vi "KI6221.vi"() -> ()   [LabVIEW 2025]
uses:
  Instance          14 14Saved   KI6221 .vi
  Instance          66 14Saved   KI6221 .vi
  Instance          40 14Saved   KI6221 .vi
  Instance          41 14Saved   KI6221 .vi
  Instance          42 14Saved   KI6221 .vi
  Instance          45 14Saved   KI6221 .vi
  Instance          50 14Saved   KI6221 .vi
  Instance          61 14Saved   KI6221 .vi
  Instance          62 14Saved   KI6221 .vi
  Instance          60 14Saved   KI6221 .vi
  Instance          68 14Saved   KI6221 .vi
  Instance          67 14Saved   KI6221 .vi
  Instance          51 14Saved   KI6221 .vi
  Instance          52 14Saved   KI6221 .vi
  Instance          53 14Saved   KI6221 .vi
  Instance          57 14Saved   KI6221 .vi
  Instance          55 14Saved   KI6221 .vi
  Instance          56 14Saved   KI6221 .vi
  Instance          54 14Saved   KI6221 .vi
  Instance          65 14Saved   KI6221 .vi
  Instance          64 14Saved   KI6221 .vi
  Instance          63 14Saved   KI6221 .vi
  Instance          37 14Saved   KI6221 .vi
  Instance          36 14Saved   KI6221 .vi
  Instance          35 14Saved   KI6221 .vi
  Instance          34 14Saved   KI6221 .vi
  Instance          39 14Saved   KI6221 .vi
  Instance          38 14Saved   KI6221 .vi
  Instance          49 14Saved   KI6221 .vi
  Instance          48 14Saved   KI6221 .vi
  Instance          43 14Saved   KI6221 .vi
  Instance          44 14Saved   KI6221 .vi
  Instance          31 14Saved   KI6221 .vi
  Instance          30 14Saved   KI6221 .vi
  Instance          32 14Saved   KI6221 .vi
  Instance          29 14Saved   KI6221 .vi
  Instance          33 14Saved   KI6221 .vi
  Instance          47 14Saved   KI6221 .vi
  Instance          26 14Saved   KI6221 .vi
  Instance          27 14Saved   KI6221 .vi
  Instance          28 14Saved   KI6221 .vi
  Instance           6 14Saved   KI6221 .vi
  Instance           5 14Saved   KI6221 .vi
  Instance           7 14Saved   KI6221 .vi
  Instance          11 14Saved   KI6221 .vi
  Instance          12 14Saved   KI6221 .vi
  Instance          13 14Saved   KI6221 .vi
  Instance          23 14Saved   KI6221 .vi
  Instance          22 14Saved   KI6221 .vi
  Instance          21 14Saved   KI6221 .vi
  Instance          20 14Saved   KI6221 .vi
  Instance          19 14Saved   KI6221 .vi
  Instance          46 14Saved   KI6221 .vi
  Instance          25 14Saved   KI6221 .vi
  Instance          18 14Saved   KI6221 .vi
  Instance          17 14Saved   KI6221 .vi
  Instance           3 14Saved   KI6221 .vi
  Instance           4 14Saved   KI6221 .vi
  Instance           2 14Saved   KI6221 .vi
  Instance          10 14Saved   KI6221 .vi
  Instance           9 14Saved   KI6221 .vi
  Instance           8 14Saved   KI6221 .vi
  <vilib>/Utility/file.llb/Write To Spreadsheet File (DBL).vi
  Instance          15 14Saved   KI6221 .vi
  Instance          16 14Saved   KI6221 .vi
  Instance          24 14Saved   KI6221 .vi
  <vilib>/express/express arith-compare/Formula/XNode/ExpressFormulaBlockNode.xnode
panel:
  in  "Case Constant\n(See Context Help) 9":bool=TRUE
  in  "Case Constant\n(See Context Help) 8":bool
  in  "Case Constant\n(See Context Help) 7":bool=TRUE
  in  "Case Constant\n(See Context Help) 6":bool=TRUE
  in  "Case Constant\n(See Context Help) 5":bool
  in  "Case Constant\n(See Context Help) 4":bool=TRUE
  in  "Case Constant\n(See Context Help) 3":bool
  in  "Case Constant\n(See Context Help) 2":bool
  in  "Case Constant\n(See Context Help)":bool=TRUE
  in  "last amp":string="*.txt"
  in  "init":bool=TRUE
  out "error out 38":errorcluster
  out "error out 37":errorcluster
  out "auto test label":string="                                                               Auto-Test Sequence Running\nThe Auto-Test sequence is attempting to locate the corresponding current levels for the voltage endpoints selected. Please be patient. If correct values can not be located, a warning window will appear. That would usually mean that either the device connections are incorrect, there is not enough signal to accurately locate the source points, or something other than the current sourced may effecting the voltage measurment."
  out "demo warning":string="DEMO MODE ON! DATA IS NOT LIVE!"
  out "INCREMENT":dbl
  in  "nv METER LAST":u16=5
  in  "enable measure LAST":bool=TRUE
  out "error out 36":errorcluster
  out "Default path 2":path=path "C:/6220software/data"
  in  "CONNECT\nONLY FLAG":bool
  in  "CAP LAST":bool
  in  "H,L,G Haz volt LAST":bool
  in  "Nearby AC voltages LAST":bool
  out "error out 35":errorcluster
  out "error out 31":errorcluster
  out "error out 22":errorcluster
  in  "Y Axis:  LAST":u16(ring)=3 items=["Points", "Time", "Current", "Voltage", "Resistance"]
  in  "X Axis: LAST":u16(ring) items=["Points", "Time", "Current", "Voltage", "Resistance"]
  out "error out 19":errorcluster
  out "error out 18":errorcluster
  in  "Source TABS LAST":u32=99
  out "error":errorcluster
  in  "Activate Output LAST":bool
  in  "Current Source \nVoltage Compliance (V) LAST":dbl=10.01 min=0.1 max=105.0 step=0.01 format="%^#_6g"
  in  "Source Level (Amps) LAST":dbl min=-0.105 max=0.105 format="%^#_9e"
  in  "SUM LAST":i32=7
  in  "NEXT FLAG LAST":i32=-1
  in  "NEXT FLAG":i32
  in  "SETUP FLAG":i32=1
  in  "Main Tabs":T1(tab)=enum."Basic Operation"
  in  "COMM\nTab Control":T2(tab)
  in  "EXIT 2":bool
  in  "conn guide":bool
  in  "SAVE 2":bool
  in  "OPEN":bool
  in  "Test file description and comments:":string="Enter details to remember about this test here. It will be saved with your test file."
  in  "EDIT present setup":bool
  in  "NEW INSTR SETUP":bool
  out "Current Test File:":path
  in  "CAP IN":u16(ring) caption="When using GUARDED CONNECTIONS we suggest that, when possible, a LO to EARTH \nConnection be made on the rear of the instrument. If this is possible given your test setup\nand goals make certain the box below is checked. If connecting instrument LO to EARTH for\nyour measurement is infeasible make certain the box below is not checked.\n         *NOTE: This response effects only how the instrument is setup. \n           Fundamentally, the measurement can be made either way." items=["NORMAL OPERATION", "REDUCE C IN 2182A"]
  in  "CANCEL":bool
  in  "BACK":bool
  out "Main intro bar":picture
  out "instrument status":string="SETUP UNVERIFIED"
  in  "Verify instruments":bool
  in  "connect HELP LINK":bool
  in  "LOW to EARTH 2":u16(ring) caption="When using GUARDED CONNECTIONS we suggest that, when possible, a LO to EARTH \nConnection be made on the rear of the instrument. If this is possible given your test setup\nand goals make certain the box below is checked. If connecting instrument LO to EARTH for\nyour measurement is infeasible make certain the box below is not checked.\n         *NOTE: This response effects only how the instrument is setup. \n           Fundamentally, the measurement can be made either way." items=["NO  EARTH  CONNECTION IN SOURCE", "LO TO EARTH CONNECTION"]
  in  "Power:":u16(ring) items=["60 Hz", "50 Hz"]
  in  "default use 2":bool
  in  "DEFAULT setup":bool=TRUE
  in  "OK":bool
  in  "HI IMP devices?":u16(ring) caption="Hi Impedance Devices also make voltage measurements more difficult. Since the input \nimpedance of the 2182 is about 10 GOhms you can approximate the 'loading error' by \ntaking your device impedance and dividing by 10^7. Therefore, if your device impedance is\n10 MOhm, then your loading error is 0.001 or 0.1%.You can compensate for this by using\nCONNECTIONS FOR HI IMPEDANCE DEVICES, however the trade off is that your noise floor\nincreases to about 100 nV RMS using this connection scheme because of the buffered input." items=["4-WIRE CONNECTIONS TO DUT", "2-WIRE CONNECTIONS TO DUT"]
  in  "6220 Connect":u16(ring)=1 caption="The current source is set up for easy cabling in STANDARD CONNECTIONS mode. This \nallows for many versatile measurement setups. However, with high impedance\ndevices or with significant cable capacitance the RC product in the circuit can impact the \ninstrument's risetime for some tests. If you would like to make GUARDED CONNECTIONS\nbecause of the RC present in your test system or for any other reason select GUARDED\nCONNECTIONS below, otherwise use STANDARD CONNECTIONS." items=["SELECT", "UNGUARDED SOURCING", "GUARDED SOURCING"]
  in  "Select GPIB Board number:\n(default to zero)":i32 min=0 max=7
  in  "Select GPIB Address number \nof the current source:":i32=16 min=0 max=32
  out "GPIB 6220 label":string="The 6220 must be connected in GPIB mode. Select the settings below."
  in  "Select Network Card number:\n(default to zero)":i32 min=0 max=7
  in  ".  IP#4":i32=160 min=0 max=255 format="%03.0f"
  in  ".  IP#3":i32=27 min=0 max=255 format="%03.0f"
  in  ".  IP#2":i32=40 min=0 max=255 format="%03.0f"
  in  "Input instrument IP Address:":i32=10 min=0 max=255 format="%03.0f"
  in  "Select the interface for the 6220/6221:":u16(ring)=1 items=["SELECT", "ETHERNET", "GPIB"]
  in  "Select the nanovoltmeter model number:":u16(ring)=3 items=["SELECT", "NONE", "2182", "2182A"]
  in  "Select the current source model number:":u16(ring)=2 items=["SELECT", "6220", "6221"]
  in  "LOW to EARTH":bool caption="When using GUARDED CONNECTIONS we suggest that, when possible, a LO to EARTH \nConnection be made on the rear of the instrument. If this is possible given your test setup\nand goals make certain the box below is checked. If connecting instrument LO to EARTH for\nyour measurement is infeasible make certain the box below is not checked.\n         *NOTE: This response effects only how the instrument is setup. \n           Fundamentally, the measurement can be made either way."
  in  "Lo earth HELP":bool
  in  "Src Connect HELP":bool
  in  "DUT connect HELP":bool
  out "WIZ string":string="Instrument Communication Setup"
  in  "NEXT":bool
  in  "nVm C HELP":bool
  in  "Previous":bool
  in  "AC HELP":bool
  in  "HAZARD HELP":bool
  in  "4 step TABS":T3(tab)
  out "step 1 pic":picture
  out "step 2 pic":picture
  out "step 3 pic":picture
  out "step 4 pic":picture
  in  "CAP":bool
  in  "H,L,G Haz volt":bool caption="I need to shield my device because:"
  in  "Nearby AC voltages":bool
  in  "start of guide":bool
  in  "END OF GUIDE":bool
  in  "NEXT GUIDE":bool
  in  "RETURN TO SPLASH SCREEN":bool
  in  "setup wizard":bool
  in  "default use":bool
  in  ".  IP#4":i32=160 min=0 max=255 format="%03.0f"
  in  ".  IP#3 2":i32=27 min=0 max=255 format="%03.0f"
  in  ".  IP#2":i32=40 min=0 max=255 format="%03.0f"
  in  "at instrument IP Address:":i32=10 min=0 max=255 format="%03.0f"
  in  "at GPIB Address:":i32=16 min=0 max=32
  in  "Model 6220 or 6221 is connected by:":u16(ring) items=["Ethernet", "GPIB"]
  in  "GPIB Address:":i32=24 min=0 max=32
  in  "INSTRUMENT NAME:":string="2400"
  in  "step setup CANCEL":bool
  in  "step setup OK":bool
  in  "DELAY in mS":i32=20 min=0
  in  "GO TO LEVEL:                *NOTE - MUST include <LEVEL>":string=":sour:volt:lev <LEVEL>"
  in  "DEACTIVATE:":string=":outp:stat off"
  in  "CONFIGURE:":string="*rst\n:sour:func volt\n:outp:stat on"
  in  "RESPONSE STRING:":string="2400"
  in  "VERIFY:":string="*IDN?"
  out "TREE DIAGRAM":picture
  out "Step source setup directions":string="Step Source Setup\nTo configure your step source correctly you must identify the GPIB commands that must be sent at each step in the testing process. The tree below defines this process. In each space to the right enter the GPIB commands that need to be sent to your stepping instrument. Each section can contain zero, one, or many commands. Each command should be separated by a Carriage Return. Do not include quotation marks or any punctuation that you do not want sent directly to the instrument. Here is a description of each step in the test:\n\nINSTRUMENT NAME - Instrument name to appear in drop down menu. This is a REQUIRED FIELD.\n\nGPIB Address - The address setting of the step source instrument.\n\nVERIFY - This section simply tests to see if the instrument responds on the bus. For Keithley Instruments this would typically be a \"*idn?\". After this section of code a READ is automatically done by the software and the response is searched to see if it includes the RESPONSE STRING. If the response string does appear, then the instrument is said to be found. If there is no response or a response without the response string, then the instrument is not found.\n\nVerify example:    *idn?\nResponse string example:   2400\n\nCONFIGURE - These commands are sent only once just after a test is executed. It should setup the instrument and activate the source at some safe level.\n\nexample:            *rst\n                           :form:elem 'volt','curr'\n                           :sour:func curr\n                           :sour:curr:rang:auto on\n                           :outp:stat on\n\nGO TO LEVEL - These commands are run once per loop. They should only set the source to the appropriate bias level for the next sweep by the 6220 and 2182. You MUST use the input variable <LEVEL> in this code. This text will be replaced with the next bias level as set from the test screen. DELAY is the time in milliseconds for the program to wait between sending these commands to the bias instrument and beginning the next 6220/2182 sweep. Use this delay to allow the bias source and device to settle before the next sweep.\n\nGO TO LEVEL example:   :sour:curr:lev <LEVEL>\n\nDEACTIVATE - These commands should be used to deactivate the step source after the last sweep. This is important for test safety.\n\nDEACTIVATE example:   :outp:stat off\n\nDATA QUERY - This is the command that tells the instrument to return data. The type of data to be returned should be set up previously in the CONFIGURE section. This is a one line command usually ending in a ?. During execution it will be immediately followed by a read which will collect the data from the instrument.\n\nDATA QUERY example:     :trac:data?\n\nNumber and Names for data Returned - Correctly fill the blank strings with names for data that will be returned. I.E. If your step source will be returning voltage and current data  enter 'Voltage' in the string when number shows 0, then click up. Now that the number reads 1 type 'Current' in the string. Make sure the strings linked to 2 and above are blank. These inputs tell the program how many different types of data it will receive as well as what to name the data vectors on data sheets and graphs. Typically, the data points are Interleaved. This means that when the instrument sends the long string of data back it would read:\n\n(Voltage,Current,Voltage,Current,....)\n\nIf this were the case you would set the data names as above.\nThen set the Data Delimiter to , \nThe Data Prefix would be (\nThe Data Suffix would be )\nand the data is interleaved so the box would be checked.\n\nAnother example:\n\nInstruments will send back:\n\nVoltage;Voltage;Voltage;.......;Current;Current;Current;\n\nIn this case set the inputs like so:\n\nNumber and Name as above.\nData Prefix:   \nData Suffix:    ;\nData Delimiter:    ;\nData is Interleaved is NOT checked because all the voltage points appear before the current values.\n\nData Prefix is left blank because nothing appears before the first number. Data Suffix is set to ; because there is a semicolon after the last data point. Data Delimiter is also set to ; because a semicolon appears between each data point.\nIf you don't wish to return any data leave the DATA QUERY blank.\n\nWhen all of your commands are correctly set click OK below. Click CANCEL to exit without saving at any time.\n"
  in  "GENERATE SCPI - BASIC":bool
  in  "Basic Source":enum32{"DC Source", "DC Sweep", "AC Source"}(tab)=enum."DC Sweep"
  in  "TAKE CONTROL":bool
  in  "Current Source \nVoltage Compliance (V)":dbl=10.01 min=0.1 max=105.0 step=0.01 format="%^#_6g"
  in  "Activate Output":bool
  in  "Source Level (Amps)":dbl min=-0.105 max=0.105 step=1e-12 format="%^#_9e"
  in  "ABORT SWEEP":bool
  in  "RUN SWEEP":bool
  in  "delta tabs 2":enum32{"GRAPH", "SHEET"}(tab)
  in  "Y Axis:":u16(ring)=3 items=["Points", "Current", "Voltage", "Resistance"]
  in  "X Axis:":u16(ring) items=["Points", "Current", "Voltage", "Resistance"]
  out "I Sweep Graph":cluster{"Y":dbl[], "Y":dbl[]}[](graph)
  out "I Sweep V Measure Data":string[][](table)
  in  "basic sweep tabs":enum32{"Source", "Measure"}(tab)
  in  "Delay (settle time in sec)":dbl=0.01 min=0.001 max=9999000.0 format="%^#_6g"
  in  "Sweep Type":u16(ring) items=["Linear ", "Logarithmic"]
  in  "Current Source \nVoltage Compliance (V)":dbl=10.0 min=0.1 max=105.0 step=0.01 format="%^#_6g"
  in  "Stop Current (Amps)":dbl=0.005 min=-0.105 max=0.105 format="%^#_6g"
  in  "Number of sweep points":i32=50 min=2 max=65536
  in  "Start Current (Amps)":dbl=0.001 min=-0.105 max=0.105 format="%^#_6g"
  in  "Measurement Integration \n(NPLCs)":dbl(ring)=1.0 items=["0.01"=0.01, "0.1"=0.1, "1"=1.0, "10"=10.0]
  in  "enable measure":bool=TRUE
  in  "Voltage Measure Range":dbl(ring)=0.1 items=["10 mV"=0.01, "100 mV"=0.1, "1 V"=1.0, "10 V"=10.0, "100 V"=100.0]
  in  "STOP 2":bool
  in  "RUN 2":bool
  in  "Voltage\n Compliance":dbl=10.0 min=0.1 max=105.0 step=0.01 format="%#_3f"
  in  "Signal Repetition \nFrequency (Hz)":dbl=10.0 min=0.0001 max=100000.0 format="%.4f"
  in  "Waveform Type":u16(ring)=1 items=["RAMP", "SQUARE", "SINE"]
  in  "waveform tabs 2":enum32{"RAMP", "SQUARE", "SINE"}(tab)=enum."SQUARE"
  in  "Duty Cycle (%)":dbl=50.0 min=0.0 max=100.0 format="%#.2f"
  in  "Ramp to: (Amps)":dbl min=-0.105 max=0.105 step=1e-12 format="%^#_6g"
  in  "Ramp from: (Amps)":dbl min=-0.105 max=0.105 step=1e-12 format="%^#.6g"
  in  "Duty Cycle (%)":dbl=50.0 min=0.0 max=100.0 format="%#.2f"
  in  "Offset (Amps)":dbl min=-0.105 max=0.105 step=1e-12 format="%^#_6g"
  in  "Amplitude (Amps)":dbl=0.105 min=0.0 max=0.105 step=1e-12 format="%^#.6g"
  in  "Offset (Amps)":dbl=0.01 min=-0.105 max=0.105 step=1e-12 format="%^#.6g"
  in  "Amplitude (Amps)":dbl=2e-12 min=2e-12 max=0.105 step=1e-12 format="%^#_6g"
  in  "GENERATE SCPI - ADVANCED":bool
  in  "Advanced Operation Tab":T4(tab)=enum."ARB Waveform Generator"
  in  "SAVE DELTA DATA":bool
  in  "CLEAR DELTA DATA":bool
  in  "delta tabs":enum32{"GRAPH", "SHEET", "HELP"}(tab)=enum."HELP"
  in  "Y Axis:":u16(ring) items=["Resistance", "Delta Voltage", "Conductance", "Power"]
  in  "X Axis:":u16(ring) items=["Points", "Time"]
  out "Delta Mode Resistance Graph":cluster{"Y":dbl[], "Y":dbl[]}[](graph)
  out "Delta Mode Measurement Data":string[][](table)
  out "Delta Measurements\nHelp":string="Delta Mode measurements are typically used on low resistance devices where noise from thermal electromotive forces becomes an issue. This software sets up an alternating current source with coordinated voltage measurements that can help to cancel out these noise sources. The inputs for this measurement are explained here:\n\nOn the Setup Tab:\n\nHigh Current (Amps) - This is the higher current value that the source will alternate between.\n\nLow Current (Amps) - This is the lower of the two alternating current values.\n\nNumber of cycles - This is the number of cycles that will be run during the test. \n\nFiltering - For Delta Mode measurements the instruments can implement either a moving filter (which averages the last X number of readings like a rolling filter) or a Repeat Filter (which only reports a result after X new readings are averaged). The number of readings is set by Filter Count. When no filter is selected Filter Count is disregarded.\n\nVoltage Measure Range - The range setting on the nanovoltmeter. A fixed range must be selected for delta mode measurements. \n\n_______________________\n\nOn the Advanced Tab:\n\nDelay (mS) - This is the delay time between the setting of the current value and the beginning of the measurement integration on the nanovoltmeter.\n\nMeasurement Integration (NPLCs) - This is the integration time for the nanovoltmeter expressed in Number of Power Line Cycles. On 60 Hz power a cycle represents 16.667 milliseconds. The lowest noise from the nanovoltmeter tends to be between 2 and 4 NPLCs for delta measurements.\n\nCurrent Source Voltage Compliance - This is the maximum potential created across the current source output leads. This should be set depending on safety and the fragility of the devices under test. This limit can be exceeded for a few microseconds until the 622X can respond. See the manual for more details.\n\nDelta Demo Mode - The demo mode button displays the demo graph for viewing example data and taking new data to show the difference between DC and Delta mode resistance measurements.\n\nAfter Run is clicked the Data Sheet and the graph will fill with data points as they are collected. The point number, delta voltage readings, the calculated resistance, the calculated conductance, the calculated power, and time stamp are all recorded. Use the X and Y Axis controls to alter the graph. Power will not be calculated if the delta is not centered around 0 (Zero DC Power)."
  out "DELTA DIAGRAM":picture
  in  "DELTA HELP LINK":bool
  in  "Guide help 3":bool
  in  "delta user tabs":enum32{"SETUP", "ADVANCED"}(tab)
  in  "Filter\nCount":i32=50 min=2 max=300
  in  "FILTER":u16(ring)=1 items=["NO Filter", "Moving Filter", "Repeat Filter"]
  in  "Voltage Measure Range":dbl(ring)=0.01 items=["10 mV"=0.01, "100 mV"=0.1, "1 V"=1.0, "10 V"=10.0, "100 V"=100.0]
  in  "INFINITE DELTA CYCLES":bool
  in  "Number of Readings":i32=1000 min=1 max=65536
  in  "Low Current (Amps)":dbl=-0.0004 min=-0.105 max=0.105 format="%^#_8e"
  in  "High Current (Amps)":dbl=0.0004 min=-0.105 max=0.105 format="%^#_8e"
  in  "DELTA DEMO":bool
  in  "DAMPING":bool
  in  "Current Source \nVoltage Compliance (V)":dbl=10.0 min=0.1 max=105.0 step=0.01 format="%^#_6g"
  in  "Measurement Integration (NPLCs)":dbl=1.0 min=1.0 max=50.0 step=1.0 format="%#_4f"
  in  "Current Source Range":dbl(ring) items=["BEST FIXED"=0.0, "100 mA"=0.1, "20 mA"=0.02, "2 mA"=0.002, "200 uA"=0.0002, "20 uA"=2e-05, "2 uA"=2e-06, "200 nA"=2e-07, "20 nA"=2e-08, "2 nA"=2e-09]
  in  "Delay (mS) - settle time":dbl=1.0 min=1.0 max=9999000.0 format="%^#_6g"
  in  "ABORT DELTA":bool
  in  "RUN DELTA":bool
  in  "DC TABS":enum32{"2-D GRAPH", "3-D PLOT", "SHEET", "HELP"}(tab)=enum."HELP"
  out "Differential Conductance Graph":cluster{"Y":dbl[], "Y":dbl[]}[](graph)
  in  "Vertical Axis:":u16(ring)=2 items=["Delta Voltage", "Resistance", "Conductance"]
  in  "Horizontal Axis:":u16(ring) items=["Voltage", "Current"]
  in  "Differential Conductance Surface Plot":refnum<k7>(container)
  in  "Plot reset":bool
  in  "Plot style":i32(ring)=5 items=["cwLine"=1, "cwPoint"=2, "cwLinePoint"=3, "cwHiddenLine"=4, "cwSurface"=5, "cwSurfaceLine"=6, "cwSurfaceNormal"=7, "cwContourLine"=8, "cwSurfaceContour"=9]
  in  "Transparency (%)":dbl(knob) scale=0.0..90.0
  in  "Projection":bool
  out "Differential Conductance Measurement Data":string[][](table)
  out "DIFF COND DIAGRAM":picture
  out "Differential Conductance \nHelp":string="Differential Conductance sweeps can be controlled in several different ways and the results examined through a number of graphs or charts.\n\nFirst, a discussion of the inputs that define a single differential conductance sweep:\n\nOn the Setup Panel:\n\nWhen controlling the sweep in terms of current these inputs appear:\n\nStart Current (Amps) - the first current value to generate a conductance reading.\n\nStop Current (Amps) - the last current value to generate a reading.\n\nNumber of sweep points - the number of points including start and stop to return values. I.E. if start is -1 nA and stop is 1 nA and number of sweep points is 21, then the first reading is taken at -1 nA, then -900 pA, -800 pA, -700 pA,.....900 pA, 1 nA.\n\nVoltage Measure Range - The range setting on the nanovoltmeter. A fixed range must be selected for Differential Conductance sweeps.\n________________________________________\n\nWhen controlling the sweep in terms of voltage these inputs appear:\n\nStart Voltage (mV) - the first voltage value to generate a conductance reading.\n\nStop Voltage (mV) - the last voltage value to generate a reading.\n\nNumber of sweep points - the number of points including start and stop to return values. I.E. if start is -1 mV and stop is 1 mV and number of sweep points is 21, then the first reading is taken at -1 mV, then -900 uV, -800 uV, -700 uV,.....900 uV, 1 mV.\n\nWhen defining the test in terms of voltage there is one other input that is enabled on the Advanced Tab. Because the test is actually being conducted by a current source and voltmeter the voltages need to be related to current. The user can select to estimate the device resistance and the instrument will convert the data points using Ohm's Law. This will work for single sweeps, but if the step source is being used to conduct multiple sweeps and create a 3-D graph, then the disadvantage is that the  start and end points may not line up appopriately as the device resistance changes at different bias points. If this is a concern then the Auto Test is recommended. Auto-Test conducts a search to find the correct voltage endpoints at the beginning of each sweep.\n\nVoltage Measure Range - This is selected automatically when controlling in voltage mode. The control will be disabled.\n\nCurrent Source Voltage Compliance - Thsi control appears on the Advanced Tab but is disabled when in voltage mode just like the Voltage Measure Range.  This is the maximum potential created across the current source output leads. This should be set depending on safety and the fragility of the devices under test. This limit can be exceeded for a few microseconds until the 622X can respond. See the manual for more details.\n_________________________________________\n\nOnly available on the Advanced Tab in Current controlled mode:\n\nCurrent Source Voltage Compliance -  This is the maximum potential created across the current source output leads. This should be set depending on safety and the fragility of the devices under test. This limit can be exceeded for a few microseconds until the 622X can respond. See the manual for more details.\n_________________________________________\n\nWhichever way you control the test these parameters must also be selected from the Advanced Tab:\n\nMeasurement Integration (NPLCs) - This is the integration time for the nanovoltmeter expressed in \nNumber of Power Line Cycles. On 60 Hz power a cycle represents 16.667 milliseconds. The lowest noise from the nanovoltmeter tends to be between 2 and 4 NPLCs for delta measurements.\n\nFiltering - For Differential Conductance measurements a Repeat Filter (which only reports a result after X new readings are averaged) can be used. The number of readings is set by Filter Count. Selecting NO Filter will disable the filter and the filter count will be ignored.\n\nDelay (settle time in mS) - this is the wait time between when the current step is made and the integration of the voltage measurement begins to allow for settling of the circuit. This is expressed in milliseconds. 1 msec is the minimum delay.\n___________________________________________\n\nFor conducting multiple differential conductance sweeps access the Step Setup Tab.\n\nEnable the step setup functions by checking the enable step source checkbox.\nOnce the step source is enabled, select start, stop, and number of step values for that source are enabled.\n\nThe Trace Offset (%Pk-Pk) control sets the y-axis offset between multiple sweeps (for the 2-D Graph), so the user can adjust how they overlap.\n\nIf the step source is disabled, one sweep will be run.\n\nUse the RUN and ABORT buttons directly below to control the test execution.\n\n"
  in  "DC HELP LINK":bool
  in  "Guide help 1":bool
  in  "DC user tabs":enum32{"SETUP", "ADVANCED", "STEP SE"}(tab)
  in  "I want to control my test in terms of:":u16(ring)=1 items=["Voltage", "Current"]
  in  "V or I DIFF CON tabs":enum32{"Voltage", "Current"}(tab)=enum."Current"
  out "voltage message":string="Voltage source compliance\nand measure range will be set automatically."
  in  "Stop Voltage (Volts)":dbl=0.1 min=-100.0 max=100.0 step=0.005 format="%^#_8g"
  in  "Number of sweep points":i32=101 min=2 max=65536
  in  "Start Voltage  (Volts)":dbl min=-100.0 max=100.0 format="%^#_8g"
  in  "Stop Current (Amps)":dbl=0.001 min=-0.105 max=0.105 format="%^#_6g"
  in  "Number of sweep points":i32=101 min=2 max=65536
  in  "Start Current (Amps)":dbl=-0.001 min=-0.105 max=0.105 format="%^#_6g"
  in  "Voltage Measure Range":dbl(ring)=0.01 items=["10 mV"=0.01, "100 mV"=0.1, "1 V"=1.0, "10 V"=10.0, "100 V"=100.0]
  in  "Delay (settle time in mS)":dbl=2.0 min=1.0 max=9999000.0 format="%^#_6g"
  in  "FILTER":u16(ring) items=["NO Filter", "Repeat Filter"]
  in  "Resistance in Ohms":dbl=100.0 min=1e-07 max=10000000000.0 format="%^#_6g"
  in  "Define source points with an:":u16(ring) items=["Auto-Test", "Estimated Resistance"]
  in  "Repeat Filter Count:":i32=2 min=2 max=300
  in  "DIFF COND DAMPING":bool
  in  "Measurement Integration (NPLCs)":dbl=1.0 min=1.0 max=50.0 step=1.0 format="%#_2f"
  in  "Current Source \nVoltage Compliance (V)":dbl=10.0 min=0.1 max=105.0 step=0.01 format="%^#_6g"
  in  "DELETE SOURCE":bool
  in  "Trace offset (% Pk-Pk):":dbl
  in  "HELP":bool
  in  "edit commands STEP SOURCE":bool
  in  "Select step source:":u16(ring) items=["2400", "Window Pop-up", "NONE", "NEW..."]
  in  "Enable \nSTEP SOURCE":bool=TRUE caption="Enable step source"
  in  "Number of steps":i32=100 min=1
  in  "Stop Level":dbl=1.0 format="%^#_3e"
  in  "Start Level":dbl format="%^#_3e"
  in  "DIFF COND SAVE DATA":bool
  in  "CLEAR DATA DIFF COND":bool
  in  "ABORT DIFF COND":bool
  in  "RUN DIFF COND":bool
  in  "PULSE user tabS":enum32{"SETUP", "TIMING", "ADVANCED"}(tab)
  in  "Voltage Measure Range":dbl(ring)=0.01 items=["10 mV"=0.01, "100 mV"=0.1, "1 V"=1.0, "10 V"=10.0, "100 V"=100.0]
  in  "Pulse Mode:":u16(ring)=1 items=["Sweep Pulse Amplitude", "Repeat Pulse Amplitude"]
  in  "PULSE SWEEP OR LEVEL TABS":enum32{"Sweep", "Repeat"}(tab)
  in  "Number of Pulses":i32=101 min=2 max=65536
  in  "Sweep Type":u16(ring) items=["Linear ", "Logarithmic"]
  in  "Stop Pulse Level (Amps)":dbl=0.05 min=-0.1 max=0.1 format="%^#_3e"
  in  "Start Pulse Level (Amps)":dbl min=-0.1 max=0.1 format="%^#_3e"
  in  "Pulse Filter Count":i32=2 min=2 max=300
  in  "PULSE FILTER":u16(ring) items=["NO Filter", "Moving Filter", "Repeat Filter"]
  in  "INFINITE REPEAT PULSE CYCLES":bool
  in  "Number of Readings":i32=100 min=1 max=65536
  in  "Pulse Level (Amps)":dbl=0.01 min=-0.105 max=0.105 format="%^#_6g"
  in  "Pulse Width (mS)":dbl=0.05 min=0.05 max=12.0 step=0.001 format="%^#.3g"
  in  "Interval between Pulses (NPLC)":dbl=5.0 min=5.0 max=999990.0 step=1.0 format="%^#_10g"
  in  "Delay - pulse settle time in mS":dbl=0.016 min=0.016 max=11.966 step=0.001 format="%^#.4g"
  in  "Number of Pulse Off Measurements":i32=2 min=0 max=2 step=1
  in  "Pulse Off Level (Amps)":dbl min=-0.105 max=0.105 format="%^#_6g"
  in  "Current Source \nVoltage Compliance (V)":dbl=10.0 min=0.1 max=105.0 step=0.01 format="%^#_3g"
  in  "pulse TABS":enum32{"GRAPH", "SHEET", "HELP"}(tab)=enum."HELP"
  in  "Y Axis:":u16(ring) items=["Resistance", "Voltage", "Conductance", "Power", "Average Power"]
  in  "X Axis:":u16(ring) items=["Points", "Current", "Time"]
  out "Pulsed IV Graph":cluster{"Y":dbl[], "Y":dbl[]}[](graph)
  out "PULSE DATA SHEET":string[][](table)
  in  "PULSE HELP BUTTON":bool
  in  "PULSE HELP TABS":enum32{"DIAGRAM 2", "DIAGRAM"}(tab)=enum."DIAGRAM"
  out "PULSE DIAGRAM-SWEEP":picture
  out "PULSE DIAGRAM":picture
  out "Pulsed IV Measurements \nHelp":string="The Model 6221 Current Source uses a special pulse mode to coordinate with the Model 2182A. These pulses can then be used to collect current and voltage data for many devices, especially those with power limitations.\n\nFrom the setup tab you can select either sweep pulse mode or repeat pulse mode. In sweep pulse mode enter the start and stop value for the pulse as well as a number of pulses and a sweep type  which set a linear or logarithmic sweep function. In repeat pulse mode set the pulse level (Amps) and the number of pulses. Set the voltage measurement range for the nanovoltmeter for the highest range you will need whether you are repeating or sweeping pulses.\n\nOn the timing tab set the pulse width (ms) and a delay - settle time (ms) for the pulse. Also, select a interval between pulses (NPLC) to wait between pulses. The  interval between pulses (NPLC) is set in Number of Power Line Cycles because the measurements each include a off level measurement before and after the pulse which are syncronized to the power line. Allowing time to sycronizing these pulses fo low voltage noise means that the minimum interval is 5 line cycles. The pulse width and interval selections determine the duty cycle. The nanovoltmeter integration time is automatically set to fill as much of the pulse as possible. The minimum integration time is 33 us, the minimum pulse width is 50 us, so the minimum pulse delay is 16 us. \n\nOn the Advanced Tab set the compliance limit for the source -  This is the maximum potential created across the current source output leads. This should be set depending on safety and the fragility of the devices under test. This limit can be exceeded for a few microseconds until the 622X can respond. See the manual for more details. This is also where to set the pulse off level (Amps). This is the value the current returns to during the pulse off times. Usually, this would only be used to negate any current offset in the source to minimize power into the device.\n\nThe voltage measurements appear in the Data Sheet and graph to the right. To save the data to a text file that can be opened in a spreadsheet editor use the Save Data button in the upper right corner.\n\nUse the RUN and ABORT buttons directly below to control the test execution."
  in  "PULSE HELP LINK":bool
  in  "Guide help 2":bool
  in  "PULSE SAVE DATA":bool
  in  "CLEAR DATA PULSE":bool
  in  "ABORT PULSE":bool
  in  "RUN PULSE":bool
  in  "Voltage\n Compliance":dbl=10.0 min=0.1 max=105.0 step=0.01 format="%#_3f"
  out "UPLOAD TIME WINDOW":string="            ARB WAVEFORM DATA UPLOAD\n\n\nDepending on the size of the complete waveform it may take a few moments to upload the data. When this window disappears, you may continue by running the waveform. The waveform will be saved in ARB1 and stored in nonvolatile memory. This\nmay take up to about 30 seconds.\n"
  out "Waveform\n Preview":dbl[](graph)=[0.0, 0.0031395259764657162, 0.006266661678215307, 0.009369065729286374, 0.012434494358242926, 0.015450849718747604, 0.018406227634234176, 0.021288964578253956, 0.02408768370508613, 0.02679133974895024, 0.029389262614624104, 0.03187119948743497, 0.034227355296434954, 0.03644843137107113, 0.03852566213879005, 0.04045084971874799, 0.042216396275101396, 0.04381533400219385, 0.04524135262330166, 0.04648882429441327, 0.04755282581475839, 0.04842915805643228, 0.04911436253643517, 0.04960573506572464, 0.049901336421414325, 0.05000000000000075, 0.04990133642141433, 0.04960573506572464, 0.04911436253643518, 0.048429158056432296, 0.04755282581475841, 0.04648882429441329, 0.04524135262330168, 0.04381533400219387, 0.042216396275101424, 0.04045084971874802, 0.03852566213879009, 0.036448431371071184, 0.034227355296435016, 0.03187119948743504, 0.02938926261462418, 0.026791339748950323, 0.024087683705086224, 0.02128896457825406, 0.018406227634234287, 0.015450849718747724, 0.012434494358243054, 0.009369065729286507, 0.006266661678215447, 0.0031395259764658624, 1.5147117501252088e-16, -0.0031395259764655597, -0.006266661678215146, -0.009369065729286209, -0.012434494358242761, -0.015450849718747436, -0.018406227634234006, -0.021288964578253782, -0.024087683705085957, -0.02679133974895007, -0.029389262614623934, -0.031871199487434804, -0.034227355296434794, -0.036448431371070976, -0.0385256621387899, -0.04045084971874785, -0.042216396275101264, -0.04381533400219372, -0.045241352623301555, -0.04648882429441318, -0.047552825814758316, -0.04842915805643222, -0.04911436253643513, -0.049605735065724604, -0.04990133642141432, -0.05000000000000075, -0.04990133642141434, -0.04960573506572466, -0.0491143625364352, -0.04842915805643232, -0.04755282581475843, -0.0464888242944133, -0.04524135262330169, -0.04381533400219386, -0.0422163962751014, -0.04045084971874798, -0.03852566213879003, -0.0364484313710711, -0.034227355296434905, -0.03187119948743491, -0.02938926261462402, -0.02679133974895014, -0.02408768370508601, -0.021288964578253813, -0.018406227634234013, -0.01545084971874742, -0.01243449435824272, -0.009369065729286143, -0.006266661678215056, -0.003139525976465444]
  in  "phaseMarker Setup":bool
  in  "ARB HELP LINK":bool
  in  "Signal Repetition \nFrequency (Hz)":dbl=10000.0 min=0.0001 max=100000.0 format="%.4f"
  in  "Graph view:":u16(ring)=1 items=["Complete waveform preview", "ScratchPad selection preview"]
  in  "Complete Waveform":i32[](listbox)=[0]
  in  "DELETE COMPLETE":bool
  in  "ADD COMPLETE":bool
  in  "INF":bool
  in  "Total Wave Duration (S)":dbl=10.0 min=0.001 format="%#_3g"
  in  "STOP":bool
  in  "RUN":bool
  in  "Save to File":bool
  in  "rename":bool
  in  "<- Compact":bool
  in  "UPLOAD":bool
  in  "DELETE SCRATCH":bool
  in  "ADD SCRATCH":bool
  in  "Waveform Type":u16(ring)=2 items=["RAMP", "SQUARE", "SINE", "DC + NOISE", "CUSTOM", "CALCULATED", "FILTER"]
  in  "waveform tabs":T5(tab)=enum."SINE"
  in  "Start Phase \n(Degrees)":dbl min=0.0 max=360.0 format="%#.3f"
  in  "Duty Cycle (%)":dbl=50.0 min=0.0 max=100.0 format="%#.2f"
  in  "Ramp to: (Amps)":dbl=0.01 min=-100.0 max=100.0 format="%^#_6g"
  in  "Ramp from: (Amps)":dbl min=-100.0 max=100.0 format="%^#.6g"
  in  "Number of Cycles":dbl=5.0 min=1.0
  in  "Number of Points per cycle":i32=20 min=1
  in  "Rise/Fall in points":i32 min=0
  in  "Start Phase \n(Degrees)":dbl min=0.0 max=360.0 format="%#.3f"
  in  "Duty Cycle (%)":dbl=50.0 min=0.0 max=100.0 format="%#.2f"
  in  "Offset (Amps)":dbl min=-100.0 max=100.0 format="%^#_6g"
  in  "Amplitude (Amps)":dbl=0.01 min=-100.0 max=100.0 format="%^#.6g"
  in  "Number of Cycles":dbl=10.0 min=1.0
  in  "Number of Points per cycle":i32=10 min=1
  in  "Start Phase \n(Degrees)":dbl min=0.0 max=360.0 format="%#.3f"
  in  "Offset (Amps)":dbl min=-100.0 max=100.0 step=1e-17 format="%^#.6g"
  in  "Amplitude (Amps)":dbl=0.05000000000000075 min=-100.0 max=100.0 step=1e-12 format="%^#_6g"
  in  "Number of Cycles":dbl=1.0 min=1.0 max=65536.0
  in  "Number of Points per cycle":i32=100 min=1 max=65536 format="%#.0f"
  in  "Offset (Amps)":dbl min=-10000000.0 max=10000000.0 format="%^#_6g"
  in  "Standard Deviation":dbl=0.01 min=0.0 max=1.0 format="%^#_6g"
  in  "Number of Cycles":dbl=1.0 min=1.0 max=65536.0
  in  "Number of Points per cycle":i32=100 min=1 max=65536 format="%#.0f"
  in  "Custom points file:":path
  in  "Constant":dbl
  in  "Scalar?":bool
  in  "math":u16(ring) items=["+", "- ", "*", "/"]
  in  "ADD 2":i32[](listbox)=[1]
  in  "ADD":i32[](listbox)=[1]
  in  "Analog filter - \nTau in # points":dbl=1.0 min=0.5 max=300000.0
  in  "filter":i32[](listbox)=[1]
  in  "ScratchPad":i32[](listbox)=[2]
  in  "milliseconds to wait":u32
  in  "BIG DISP Ohm Overlay":bool caption="W"
  in  "SEND COMM":bool
  in  "Command String":string
  in  "RESET":bool
  in  "virtual front panel HELP LINK":bool
  in  "______________________________________________________________________________________________________________":bool
  in  "BIG DISP OVERLAY":bool
  in  "LITTLE DISP OVERLAY":bool
  in  "CONTROL":bool
  out "LIGHT":bool
  in  "CURSOR RIGHT":bool
  in  "CURSOR LEFT":bool
  in  "OUTPUT":bool
  in  "RANGE AUTO":bool
  in  "RANGE DOWN":bool
  in  "RANGE UP":bool
  in  "ENTER":bool
  in  "EXIT":bool
  in  "MENU":bool
  in  "knob push":bool
  in  "NUM+/-":bool
  in  "AVG":bool
  in  "TRIAX":bool
  in  "SETUP":bool
  in  "SAVE":bool
  in  "FREQ":bool
  in  "AMPL":bool
  in  "RECALL":bool
  in  "UNITS":bool
  in  "TRIG":bool
  in  "DISP":bool
  in  "ADDR":bool
  in  "COMM":bool
  in  "WAVE":bool
  in  "PULSE":bool
  in  "DELTA":bool
  in  "COND":bool
  in  "SWP":bool
  in  "DC":bool
  in  "PRES":bool
  in  "FILTER 2":bool
  in  "config":bool
  in  "local":bool
  in  "Knob":i16(knob) scale=0.0..10.0
  out "SUB READING 6220":string="Compliance: 010.00 V            "
  out "MAIN 6220 READING":string="+00.000 mA      OFF "
  out "FRONT PANEL 6220":picture
  out "HELP TEXT":string="This software package is distributed by Keithley Instruments for use with the Model 6220 or Model 6221 DC and AC Current Source and the Model 2182A Nanovoltmeter. If you experience problems or have questions regarding this software please go to www.keithley.com or click the link above. Then click on contact us to submit questions to our applications department. You can also reach us toll free at 800-552-1115. \n\nWEB UPDATES above direct you to download the latest update to this software.\n\nDEMO MODE enables or disables Demo Mode. When the button is dark gray demo mode is enabled and live instrument communication does not take place.\n"
  in  "DEMO MODE":bool
  in  "connect HELP LINK 2":bool
  out "WEB UPDATE STR":string="We are connecting to the Keithley Web Update service. Please be patient..."
  out "debug str":string="We are sending Bug/Feedback information. Please be Patient..."
  in  "WEB UPDATES":bool
  in  "MAIN HELP LINK":bool
  in  "APPS":bool
  in  "user's web":bool
  in  "www":bool
  in  "BUG REPORT":bool
  out "error out":errorcluster
  out "Setup String":string=":SYST:COMM:SERIal:SEND \"SYST:FFIL ON\"\r\n:OUTP:ISH OLOW\r\n:outp:lte OFF"
  in  "COMM TAB LAST":u32=5
  in  "4 step TABS LAST":i32=3
  out "error out 3":errorcluster
  in  "Measure Connect LAST":u16=5
  in  "LOW2EARTH LAST":u16
  in  "6220 Connect LAST":u16=1
  out "error out 9":errorcluster
  out "error out 11":errorcluster
  out "error out 34":errorcluster
  out "error out 33":errorcluster
  out "error out 32":errorcluster
  out "error out 29":errorcluster
  in  "STEP SOURCE LAST":i32
  in  "OFFSET DC LAST":dbl
  out "error out 30":errorcluster
  out "error out 28":errorcluster
  out "error out 27":errorcluster
  out "error out 26":errorcluster
  in  "DATA .H":string="The DATA code queries the Model 6220/6221 for the contents of the buffer. When you see ENTER100000 this indicates you need to read data from the box. The number is the recommended number of bytes to read. This depends on how many buffer points were filled. This command selects a starting point \"0\" and a number of buffer points to download \"<DATACOUNT>\"."
  in  "STOP ARB .H":string="The STOP ARB code aborts any waveform that is running, then turns off the output. "
  in  "ABORT .H":string="The ABORT code aborts any sweep or measurements running. It can also be a good idea to turn off the output or reset the instruments to its defaults when aborting a test."
